vi "MeasureSignals.vi"(6 "Path":path, 8 "error in (no error)":errorcluster caption="Error in", 11 "DevicesAndSignals":T1) -> (0 "error out":errorcluster caption="Error out", 3 "DevicesAndSignals":T1)   [LabVIEW 2016]
doc: "Use this VI to interactively choose signals you want to measure and visualize or save.\n\nDevicesAndSignals: Cluster consisting of an array of devices and an array of all signals you want to measure\nPath: Complete path and name of the file to save measurement values in."
uses:
  <vilib>/Utility/error.llb/DialogType.ctl
panel:
  in  "cmdSaveOnOff":bool
  out "lbDataFile":string
  in  "cmdExit":bool
  in  "Signals":i32(listbox)
  out "Signalverlaufsdiagramm":waveform(dbl)[](graph)
  in  "cmdStop":bool
  in  "cmdStart":bool
  # "Save measurement data"
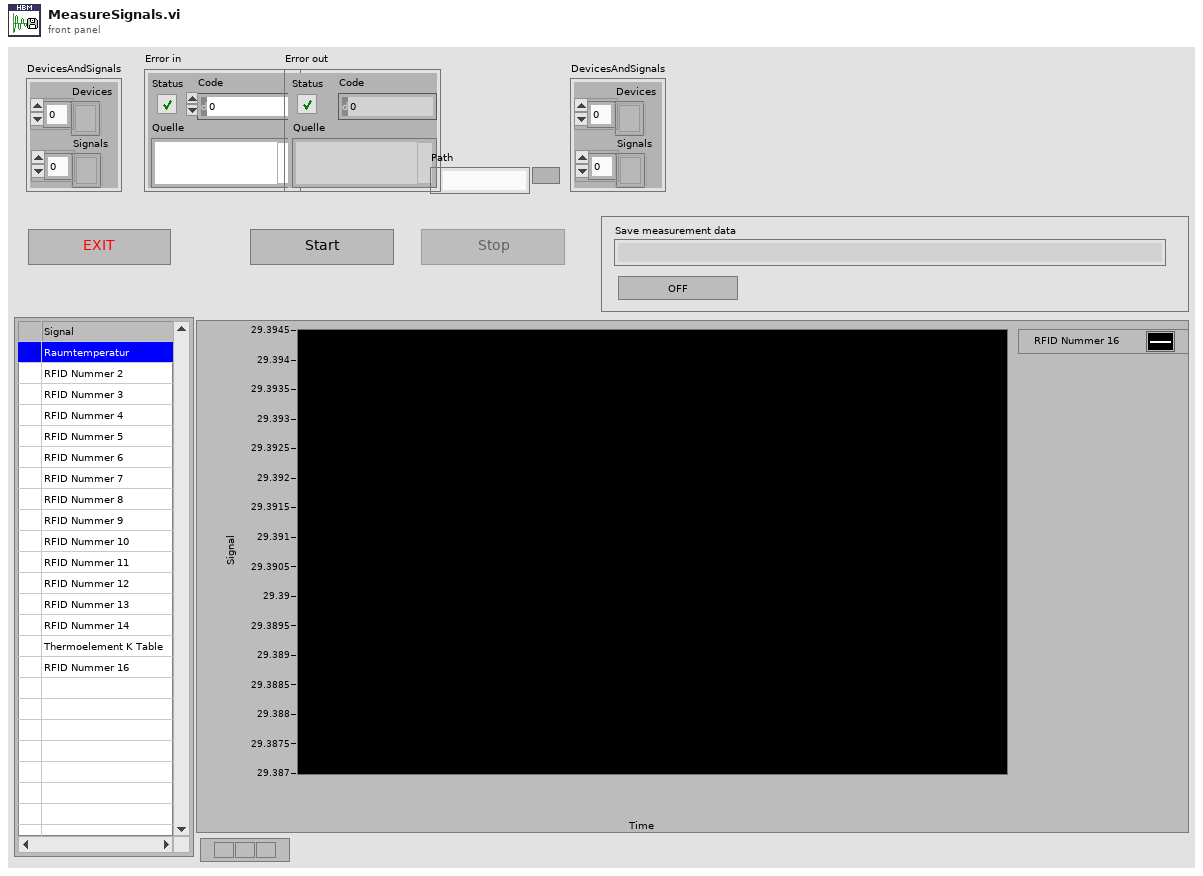
[diagram p1: front panel]
types:
  T1 = cluster{"Devices":refnum<k24>[], "Signals":refnum<k24>[]}
  T2 = enum16{"open", "open or create", "create or replace", "create", "open (read-only)"}
  T3 = cluster{"MeasData":waveform(dbl)[], "State":enum16{"Data", "Exit"}}
  T4 = enum16{"Initialize", "Exit", "DAQ_Start", "DAQ_Stop"}
  T5 = enum16{"Idle", "DAQ_Initialize", "DAQ_Start", "DAQ_Read", "DAQ_Stop", "Exit"}
  T6 = typedef "DialogType.ctl" = u16
  T7 = enum8{"Enabled", "Disabled", "Disabled and Grayed Out"}
  T8 = typedef "LVPoint32TypeDef.ctl" = cluster{"Horizontal":i32, "Vertical":i32}
  T9 = typedef "LVRowAndColumnTypeDef.ctl" = cluster{"Row":i32, "Column":i32}
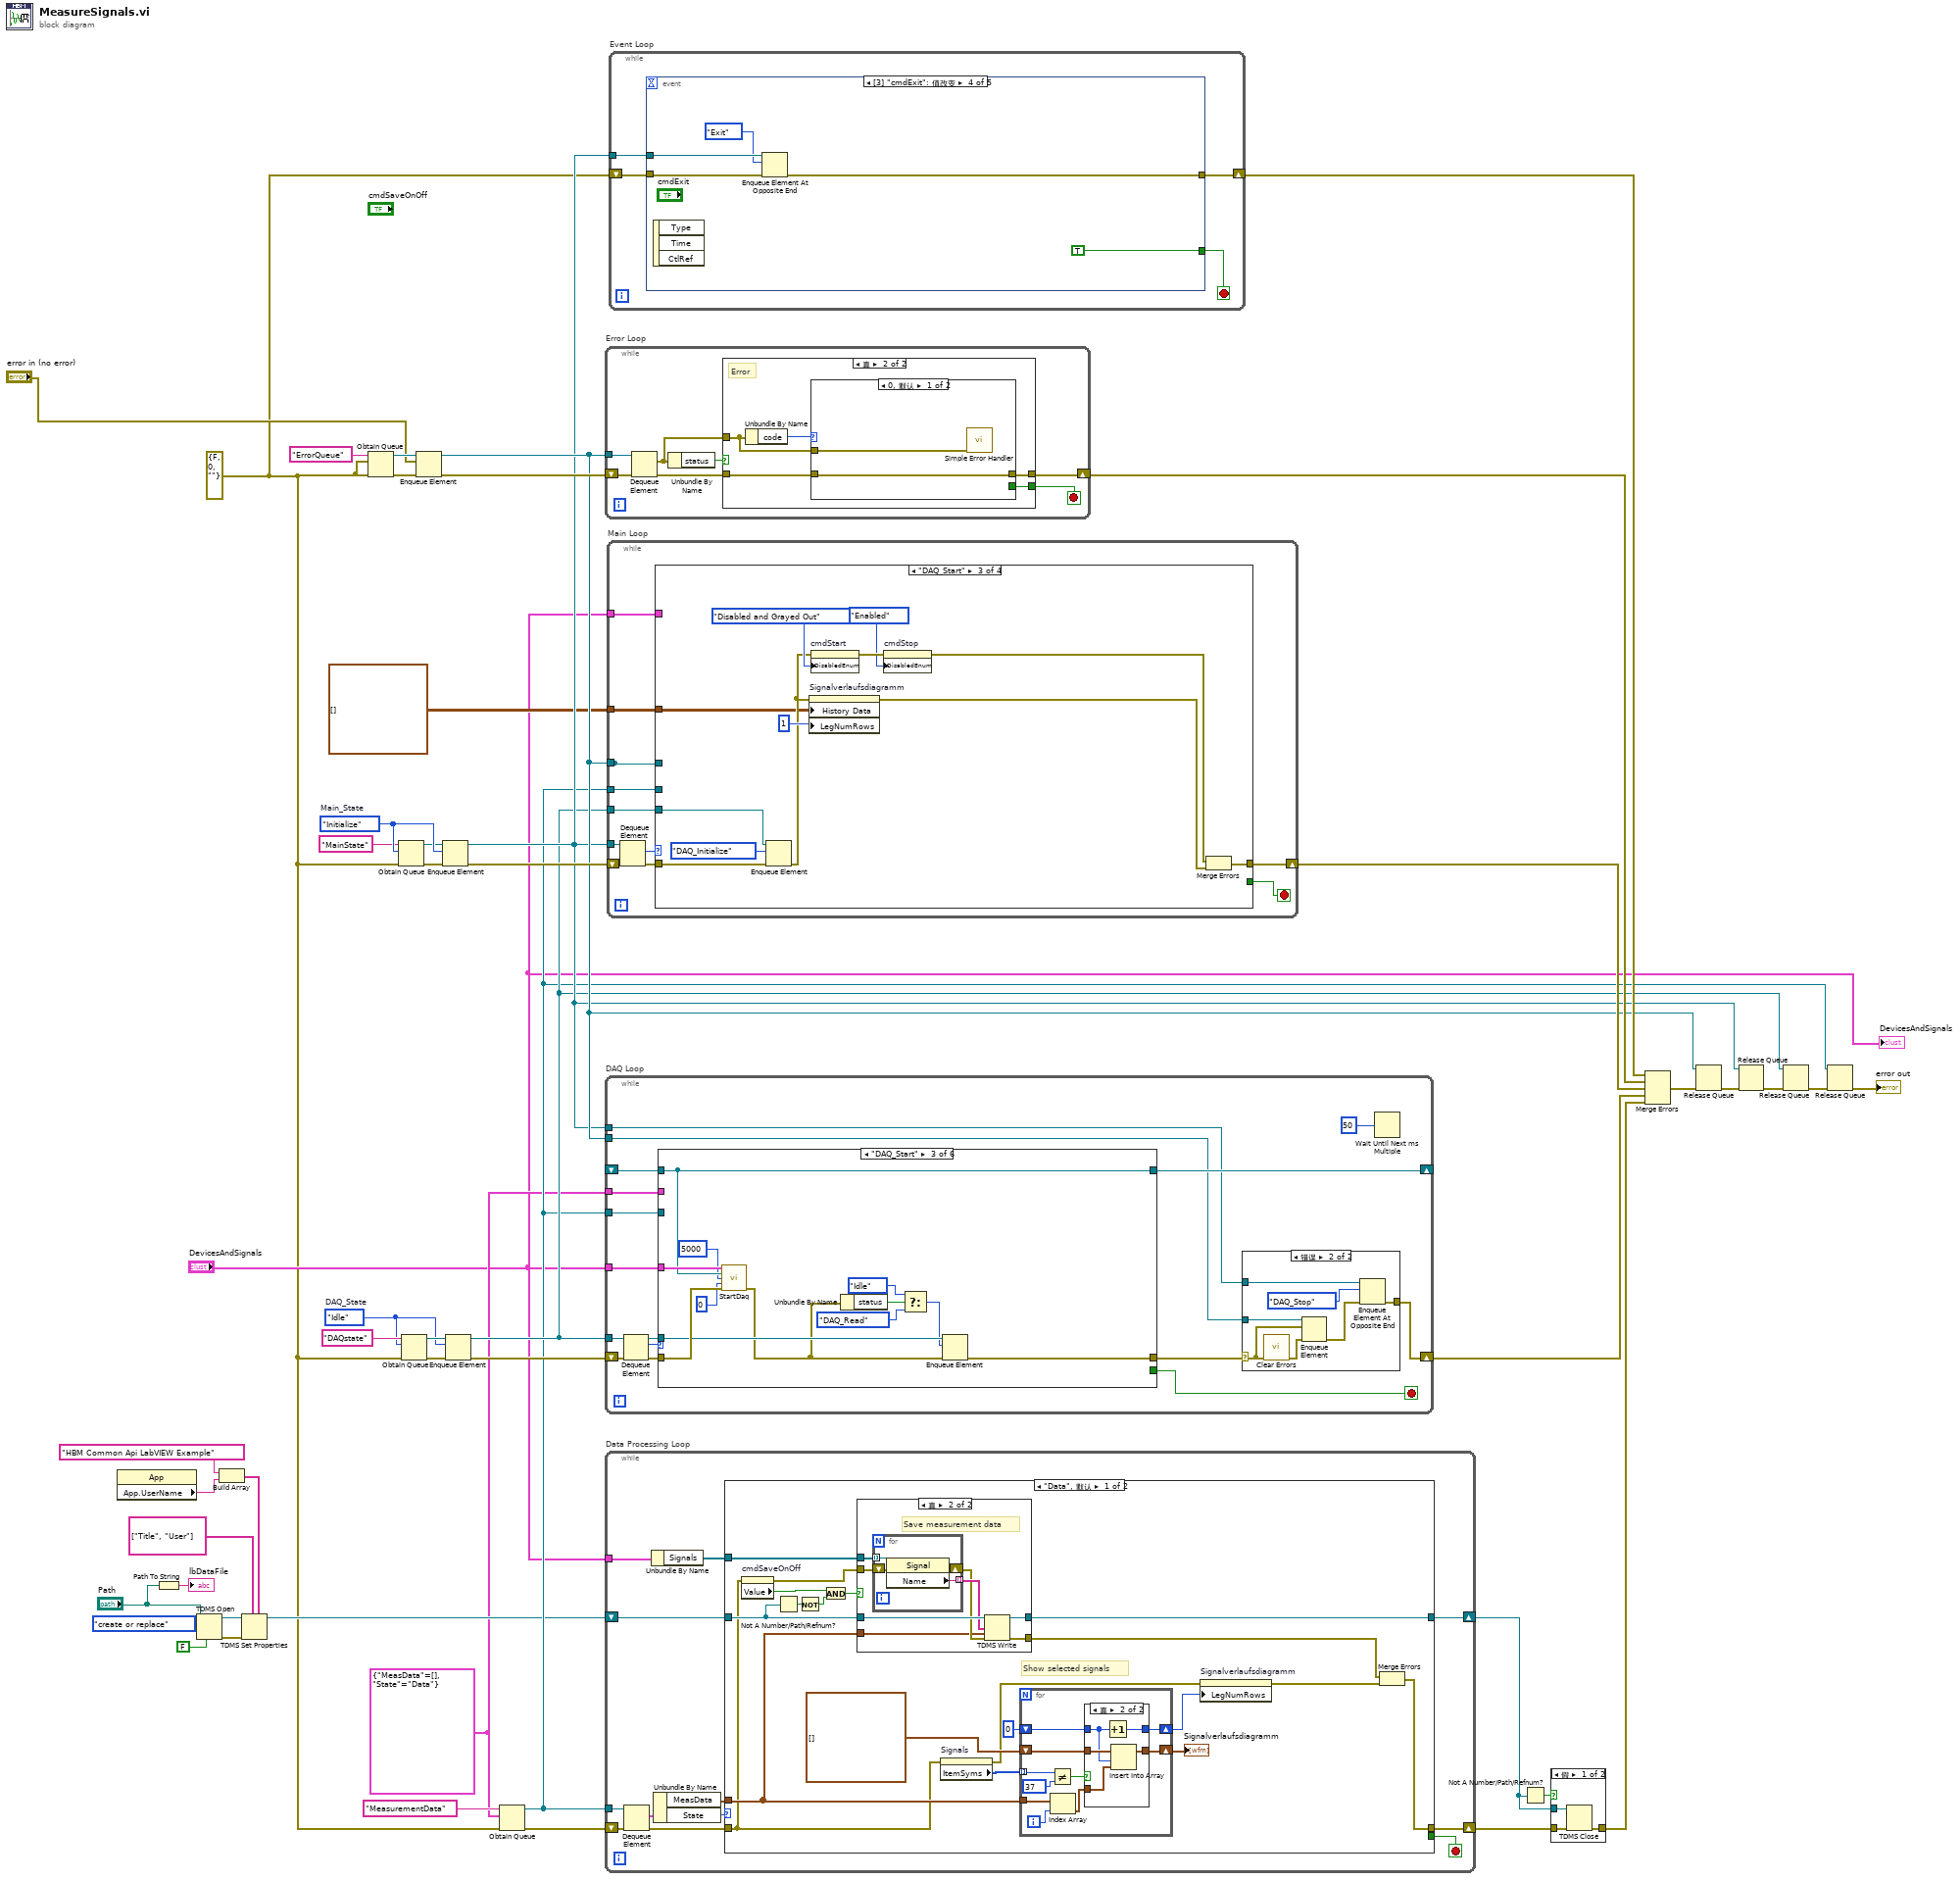
[diagram p0: block diagram]
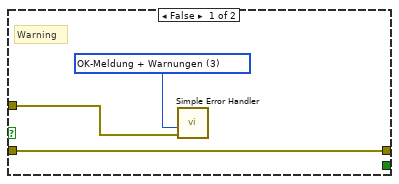
[diagram p3: hidden frame]
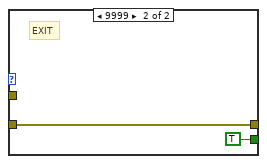
[diagram p4: hidden frame]
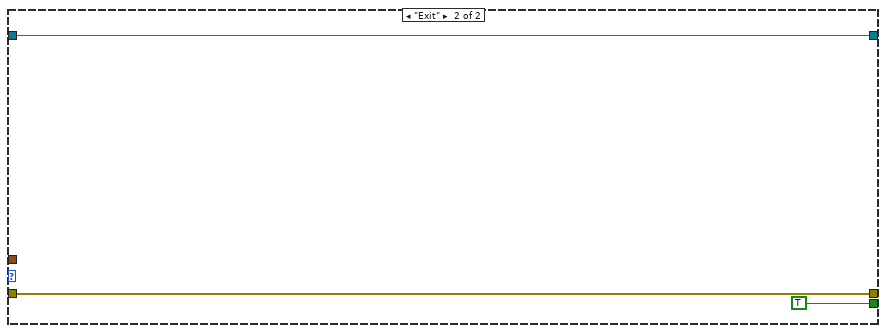
[diagram p7: hidden frame]
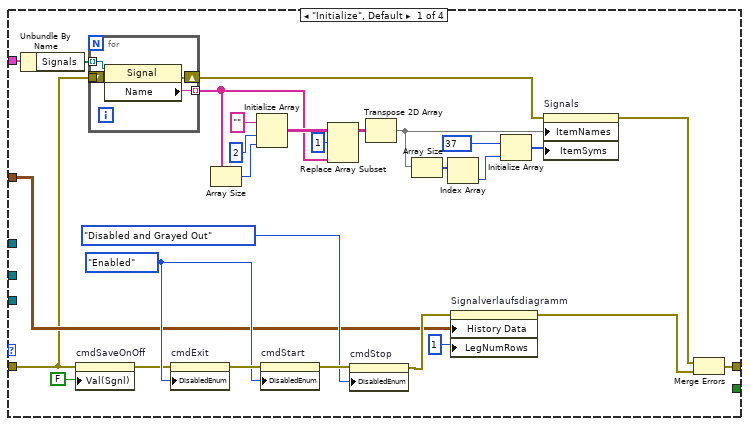
[diagram p8: hidden frame]
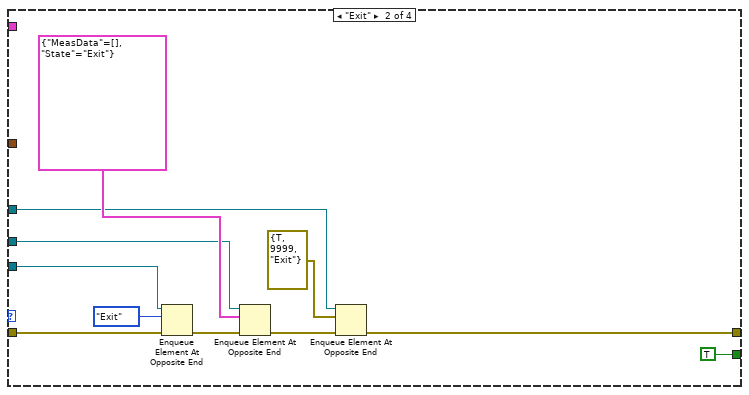
[diagram p9: hidden frame]
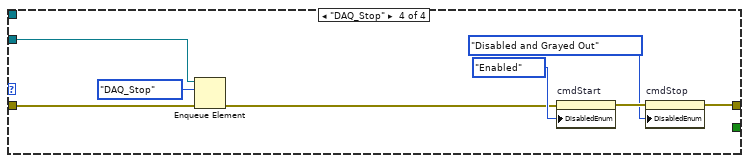
[diagram p10: hidden frame]
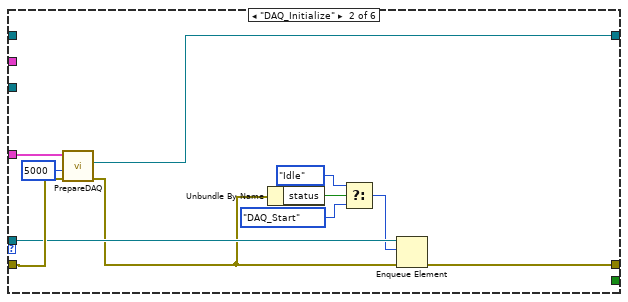
[diagram p13: hidden frame]
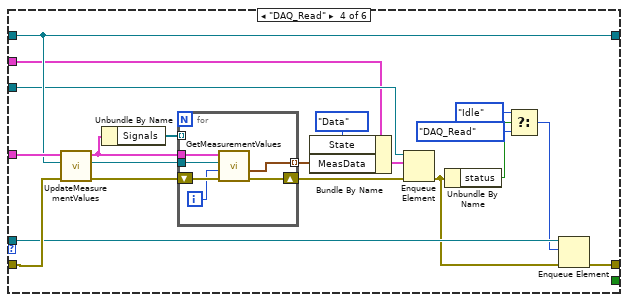
[diagram p14: hidden frame]
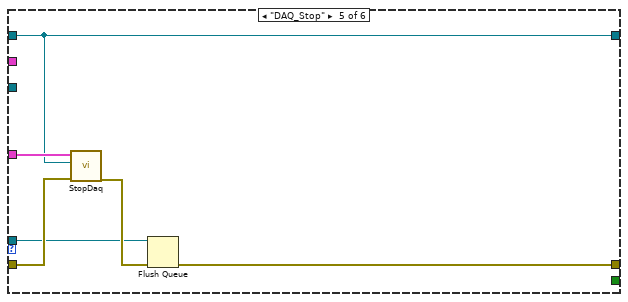
[diagram p15: hidden frame]
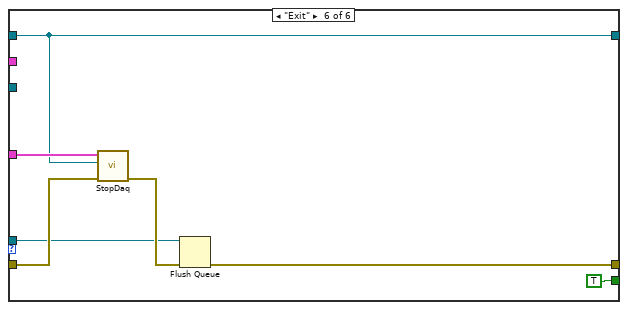
[diagram p16: hidden frame]
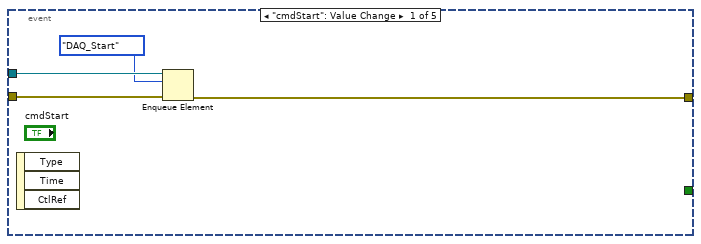
[diagram p17: hidden frame]
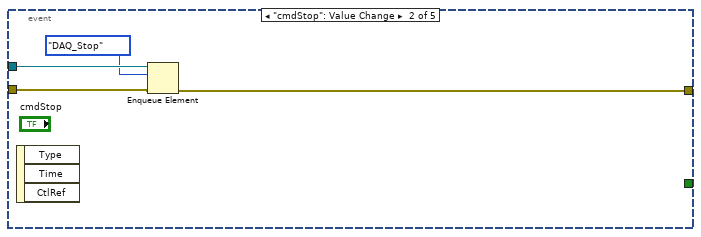
[diagram p18: hidden frame]
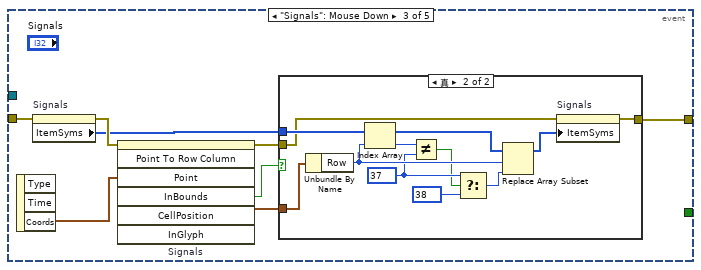
[diagram p19: hidden frame]
diagram:
  w1 = errorcluster {"status"=FALSE, "code"=0, "source"=""} ("Fehler (Eingang, kein Fehler)")
  w11 = T3 {"MeasData"=[], "State"=enum."Data"} ("Element")
  w45 = T4."Initialize"  # Main_State
  w46 = T5."Idle"  # DAQ_State
  n1 = property class="App"() -> ("App.UserName"=w17:string)  [unwired: 2 in, 2 out]
  n2 = Path To String(path="Path") -> (string=→"lbDataFile":string)
  n3 = TDMS Open(6:FALSE ("Pufferung deaktivieren? (T)"), 10:T2."create or replace" ("Operation (0:Öffnen)"), 11:"Path") -> (0:w19:errorcluster, 3:w13:refnum<k34>)  [unwired: 4 in]
  n4 = Build Array("HBM Common Api LabVIEW Example", w17) -> (w16:string[])
  n5 = TDMS Set Properties(5:w16, 7:string[] ["Title", "User"] ("property names"), 8:w19, 11:w13) -> (3:w12:refnum<k34>)  [unwired: 2 in, 3 out]
  n6 = Obtain Queue(name (unnamed)="ErrorQueue" ("Name (unbenannt)"), element data type=w1, error in (no error)=w1) -> (queue out=w37:refnum<queue>, error out=w38:errorcluster)  [unwired: 2 in, 1 out]
  n7 = Obtain Queue(name (unnamed)="MainState" ("Name (unbenannt)"), element data type=w45, error in (no error)=w1) -> (queue out=w44:refnum<queue>, error out=w43:errorcluster)  [unwired: 2 in, 1 out]
  n8 = Obtain Queue(name (unnamed)="DAQstate" ("Name (unbenannt)"), element data type=w46, error in (no error)=w1) -> (queue out=w47:refnum<queue>, error out=w48:errorcluster)  [unwired: 2 in, 1 out]
  n9 = Enqueue Element(queue=w37, element="error in (no error)", error in (no error)=w38) -> (queue out=w24:refnum<queue>, error out=w36:errorcluster)  [unwired: 1 in, 1 out]
  n10 = Enqueue Element(queue=w44, element=w45, error in (no error)=w43) -> (queue out=w23:refnum<queue>, error out=w41:errorcluster)  [unwired: 1 in, 1 out]
  n11 = Enqueue Element(queue=w47, element=w46, error in (no error)=w48) -> (queue out=w22:refnum<queue>, error out=w35:errorcluster)  [unwired: 1 in, 1 out]
  n12 = Obtain Queue(name (unnamed)="MeasurementData" ("Name (unbenannt)"), element data type=w11, error in (no error)=w1) -> (queue out=w21:refnum<queue>, error out=w34:errorcluster)  [unwired: 2 in, 1 out]
  n13 = while "Error Loop" {
    tunnel: w24 -> [w56]
    shift-right: [w50] -> w32
    shift-left: w36 -> [w52]
    stop <- w53 stop-if-true
    n14 = Dequeue Element(queue=w56, error in (no error)=w52) -> (element=w54:errorcluster, error out=w51:errorcluster)  [unwired: 1 in, 2 out]
    n15 = Unbundle By Name(w54) -> ("status"=w55:bool)
    n16 = case "Case-Struktur" shown="真" w55 {
      tunnel: w54 -> [w59 w62]
      tunnel: [_ w63] -> w53
      tunnel: w51 -> [w57 w61]
      tunnel: [w57 w60] -> w50
      frame False {
        w58 = T6 3 items=["Kein Dialog", "OK-Meldung", "Dialog zum Fortsetzen oder Anhalten", "OK-Meldung + Warnungen", "Weiter/Stopp + Warnung"] ("type of dialog (OK msg:1)")
        # "Warning"
        n17 = call <vilib>:"Simple Error Handler.vi"("type of dialog (OK msg:1)"=w58, "error in (no error)"=w59) -> ()  [unwired: 3 in, 5 out]
      }
      frame True {
        # "Error"
        n18 = Unbundle By Name(w62) -> ("code"=w64:i32)
        n19 = case shown="0, 默认" w64 {
          tunnel: [_ TRUE] -> w63
          tunnel: w62 -> [w66 _]
          tunnel: w61 -> [w65 w67]
          tunnel: [w65 w67] -> w60
          frame 0, Default {
            n20 = call <vilib>:"Simple Error Handler.vi"("error in (no error)"=w66) -> ()  [unwired: 4 in, 5 out]
          }
          frame 9999 {
            # "EXIT"
          }
        }
      }
    }
  }
  n21 = while "DAQ Loop" {
    tunnel: w22 -> [w84]
    tunnel: "DevicesAndSignals" -> [w82]
    shift-right: [w81] -> _
    shift-left: _ -> [w78]
    shift-right: [w72] -> w30
    shift-left: w35 -> [w80]
    tunnel: w21 -> [w75]
    tunnel: w11 -> [w74]
    tunnel: w24 -> [w73]
    tunnel: w23 -> [w71]
    stop <- w76 stop-if-true
    n22 = Dequeue Element(queue=w84, error in (no error)=w80) -> (queue out=w77:refnum<queue>, element=w83:T5, error out=w79:errorcluster)  [unwired: 1 in, 1 out]
    n23 = case shown="\"DAQ_Start\"" w83 {
      tunnel: w82 -> [_ w105 w117 w137 w148 w156]
      tunnel: [w94 w103 w116 w131 w144 w150] -> w81
      tunnel: w79 -> [w93 w104 w115 w132 w149 w155]
      tunnel: w78 -> [w94 _ w116 w131 w144 w150]
      tunnel: [w93 w98 w113 w122 w147 w151] -> w69
      tunnel: w77 -> [_ w99 w114 w121 w145 w152]
      tunnel: [_ _ _ _ _ TRUE] -> w76
      tunnel: w75 -> [_ _ _ w129 _ _]
      tunnel: w74 -> [_ _ _ w128 _ _]
      frame "Idle", Default {
      }
      frame "DAQ_Initialize" {
        n24 = call "PrepareDAQ.vi"("Error in"=w104, "BufferTimeout"=5000, "DevicesAndSignals"=w105) -> ("Error out"=w97:errorcluster, "DaqMeasurement"=w103:refnum<k24>)  [unwired: 6 in, 1 out]
        n25 = Unbundle By Name(w97) -> ("status"=w100:bool)
        n26 = Select(t=T5."Idle" ("Element"), s=w100, f=T5."DAQ_Start" ("Element")) -> (s? t:f=w96:T5)
        n27 = Enqueue Element(queue=w99, element=w96, error in (no error)=w97) -> (error out=w98:errorcluster)  [unwired: 1 in, 2 out]
      }
      frame "DAQ_Start" {
        n28 = call "StartDaq.vi"("DevicesAndSignals"=w117, "DaqMeasurement"=w116, "SyncTimeout"=5000, "AcquisitionMode"=0, "Error in"=w115) -> ("Error out"=w108:errorcluster)  [unwired: 7 in, 3 out]
        n29 = Unbundle By Name(w108) -> ("status"=w110:bool)
        n30 = Select(t=T5."Idle" ("Element"), s=w110, f=T5."DAQ_Read" ("Element")) -> (s? t:f=w109:T5)
        n31 = Enqueue Element(queue=w114, element=w109, error in (no error)=w108) -> (error out=w113:errorcluster)  [unwired: 1 in, 2 out]
      }
      frame "DAQ_Read" {
        n32 = call "UpdateMeasurementValues.vi"("Error in"=w132, "DaqMeasurement"=w131, "DevicesAndSignals"=w137) -> ("Error out"=w135:errorcluster, "DaqMeasurement"=w136:refnum<k24>, "DevicesAndSignals"=w134:T1)  [unwired: 6 in]
        n33 = Unbundle By Name(w134) -> ("Signals"=w133:refnum<k24>[])
        n34 = for {
          tunnel: w134 -> [w143]
          tunnel: w136 -> [w142]
          shift-right: [w141] -> w130
          shift-left: w135 -> [w140]
          tunnel: w133 -> [_] mode=indexing
          tunnel: [w138] -> w126 mode=indexing
          i -> [w139]
          n35 = call "GetMeasurementValues.vi"("Error in"=w140, "Index"=w139, "DaqMeasurement"=w142, "DevicesAndSignals"=w143) -> ("Error out"=w141:errorcluster, "Waveform"=w138:waveform(dbl))  [unwired: 4 in, 2 out]
        }
        n36 = Bundle By Name(cluster=w128, "State"=enum16{"Data", "Exit"}."Data", "MeasData"=w126) -> (w127:T3)
        n37 = Enqueue Element(queue=w129, element=w127, error in (no error)=w130) -> (error out=w118:errorcluster)  [unwired: 1 in, 2 out]
        n38 = Unbundle By Name(w118) -> ("status"=w119:bool)
        n39 = Select(t=T5."Idle" ("Element"), s=w119, f=T5."DAQ_Read" ("Element")) -> (s? t:f=w120:T5)
        n40 = Enqueue Element(queue=w121, element=w120, error in (no error)=w118) -> (error out=w122:errorcluster)  [unwired: 1 in, 2 out]
      }
      frame "DAQ_Stop" {
        n41 = call "StopDaq.vi"("Error in"=w149, "DaqMeasurement"=w144, "DevicesAndSignals"=w148) -> ("Error out"=w146:errorcluster)  [unwired: 7 in, 1 out]
        n42 = Flush Queue(queue=w145, error in (no error)=w146) -> (error out=w147:errorcluster)  [unwired: 2 out]
      }
      frame "Exit" {
        n43 = call "StopDaq.vi"("Error in"=w155, "DaqMeasurement"=w150, "DevicesAndSignals"=w156) -> ("Error out"=w153:errorcluster)  [unwired: 7 in, 1 out]
        n44 = Flush Queue(queue=w152, error in (no error)=w153) -> (error out=w151:errorcluster)  [unwired: 2 out]
      }
    }
    n45 = case shown="错误" w69 {
      selector: w69 -> [w85 w86]
      tunnel: w73 -> [_ w92]
      tunnel: [w85 w88] -> w72
      tunnel: w71 -> [_ w90]
      frame No Error {
      }
      frame Error {
        n46 = call <vilib>:"Clear Errors.vi"("error in (no error)"=w86) -> ("error out"=w91:errorcluster)  [unwired: 5 in, 1 out]
        n47 = Enqueue Element(queue=w92, element=w86, error in (no error)=w91) -> (error out=w89:errorcluster)  [unwired: 1 in, 2 out]
        n48 = Enqueue Element At Opposite End(queue=w90, element=T4."DAQ_Stop" ("Element"), error in (no error)=w89) -> (error out=w88:errorcluster)  [unwired: 1 in, 2 out]
      }
    }
    n49 = Wait Until Next ms Multiple(millisecond multiple=u32 50 ("Vielfache von ms")) -> ()  [unwired: 1 out]
  }
  n50 = while "Data Processing Loop" {
    tunnel: "DevicesAndSignals" -> [w160]
    tunnel: w21 -> [w168]
    shift-right: [w163] -> w5
    shift-left: w34 -> [w165]
    shift-right: [w161] -> w7
    shift-left: w12 -> [w162]
    stop <- w166 stop-if-true
    n51 = Dequeue Element(queue=w168, error in (no error)=w165) -> (element=w158:T3, error out=w164:errorcluster)  [unwired: 1 in, 2 out]
    n52 = Unbundle By Name(w160) -> ("Signals"=w159:refnum<k24>[])
    n53 = Unbundle By Name(w158) -> ("MeasData"=w157:waveform(dbl)[], "State"=w167:enum16{"Data", "Exit"})
    n54 = case shown="\"Data\", 默认" w167 {
      tunnel: [_ TRUE] -> w166
      tunnel: w164 -> [w171 w220]
      tunnel: [w173 w220] -> w163
      tunnel: w162 -> [w178 w219]
      tunnel: [w187 w219] -> w161
      tunnel: w159 -> [w181 _]
      tunnel: w157 -> [w180 _]
      frame "Data", Default {
        # "Show selected signals"
        n55 = property on="cmdSaveOnOff" class="Bool (严格)"(error in=w171) -> (error out=w170:errorcluster, "Value"=w169:bool)  [unwired: 1 in, 1 out]
        n56 = Not A Number/Path/Refnum?(number/path/refnum=w178) -> (NaN/Path/Refnum?=w177:bool)
        n57 = Not(x=w177) -> (.not. x?=w176:bool)
        n58 = And(x=w169, y=w176) -> (x .and. y?=w175:bool)
        n59 = case "Case-Struktur" shown="真" w175 {
          tunnel: w178 -> [w189 w197]
          tunnel: [w189 w196] -> w187
          tunnel: w181 -> [_ w193]
          tunnel: w180 -> [_ w192]
          tunnel: w170 -> [w188 w191]
          tunnel: [w188 w190] -> w174
          frame False {
          }
          frame True {
            # "Save measurement data"
            n60 = for {
              tunnel: w193 -> [w201] mode=indexing
              tunnel: [w200] -> w195 mode=indexing
              shift-right: [w198] -> w194
              shift-left: w191 -> [w199]
              n61 = property on="Eigenschaftsknoten" class="Signal"(reference=w201, error in=w199) -> (error out=w198:errorcluster, "Name"=w200:string)  [unwired: 1 out]
            }
            n62 = TDMS Write(0:w197, 7:w195, 9:w192, 11:w194) -> (4:w196:refnum<k34>, 15:w190:errorcluster)  [unwired: 2 in, 2 out]
          }
        }
        n63 = property on="Signals" class="MCListbox (严格)"(error in=w171) -> (error out=w179:errorcluster, "ItemSyms"=w186:i32[])  [unwired: 1 in, 1 out]
        n64 = for {
          tunnel: w180 -> [w211]
          tunnel: w186 -> [w209] mode=indexing
          shift-right: [w205] -> w183
          shift-left: waveform(dbl)[] [] -> [w204]
          shift-right: [w202] -> w182
          shift-left: u32 0 -> [w203]
          i -> [w208]
          n65 = Not Equal?(x=w209, y=37) -> (x != y?=w206:bool)
          n66 = Index Array(array=w211, index=w208) -> (element=w207:waveform(dbl))
          n67 = case shown="真" w206 {
            tunnel: [w213 w218] -> w205
            tunnel: w204 -> [w213 w217]
            tunnel: [w212 w215] -> w202
            tunnel: w207 -> [_ w216]
            tunnel: w203 -> [w212 w214]
            frame False {
            }
            frame True {
              n68 = Increment(x=w214) -> (x+1=w215:u32)
              n69 = Insert Into Array(array=w217, index=w214, new element=w216) -> (w218:waveform(dbl)[])
            }
          }
        }
        "Signalverlaufsdiagramm" <- w183
        n70 = property on="Signalverlaufsdiagramm" class="WFChart (严格)"(error in=w179, "LegNumRows"=w182) -> (error out=w172:errorcluster)  [unwired: 1 in, 1 out]
        n71 = Merge Errors(w174, w172) -> (w173:errorcluster)
      }
      frame "Exit" {
      }
    }
  }
  n72 = while "Main Loop" {
    shift-right: [w226] -> w33
    shift-left: w41 -> [w232]
    tunnel: w23 -> [w231]
    tunnel: w22 -> [w228]
    tunnel: w21 -> [w225]
    tunnel: [w224] -> _
    tunnel: w24 -> [w224]
    tunnel: "DevicesAndSignals" -> [w223]
    tunnel: waveform(dbl)[][] [] ("Historiendaten") -> [w222]
    stop <- w227 stop-if-true
    n73 = Dequeue Element(queue=w231, error in (no error)=w232) -> (element=w230:T4, error out=w229:errorcluster)  [unwired: 1 in, 2 out]
    n74 = case shown="\"DAQ_Start\"" w230 {
      tunnel: w229 -> [w235 w273 w286 w294]
      tunnel: w228 -> [_ w274 w285 w293]
      tunnel: [_ TRUE _ _] -> w227
      tunnel: [w241 w266 w279 w289] -> w226
      tunnel: w225 -> [_ w270 _ _]
      tunnel: w224 -> [_ w268 _ _]
      tunnel: w223 -> [w256 _ _ _]
      tunnel: w222 -> [w237 _ w276 _]
      frame "Initialize", Default {
        w258 = T7."Enabled" ("Deaktiviert")
        n75 = Unbundle By Name(w256) -> ("Signals"=w255:refnum<k24>[])
        n76 = property on="cmdSaveOnOff" class="Bool (严格)"(error in=w235, "Val(Sgnl)"=FALSE ("Wert (signalisierend)")) -> (error out=w234:errorcluster)  [unwired: 1 in, 1 out]
        n77 = for {
          tunnel: [w264] -> w245 mode=indexing
          tunnel: w235 -> [w263]
          tunnel: w255 -> [w262] mode=indexing
          shift-right: [w261] -> w242
          shift-left: _ -> [_]
          n78 = property on="Eigenschaftsknoten" class="Signal"(reference=w262, error in=w263) -> (error out=w261:errorcluster, "Name"=w264:string)  [unwired: 1 out]
        }
        n79 = property on="cmdExit" class="Bool"(error in=w234, "DisabledEnum"=w258) -> (error out=w260:errorcluster)  [unwired: 1 in, 1 out]
        n80 = Array Size(array=w245) -> (size(s)=w249:i32)
        n81 = Initialize Array("" ("Element"), 2 ("Dimension"), w249) -> (w253:string[][])
        n82 = property on="cmdStart" class="Bool"(error in=w260, "DisabledEnum"=w258) -> (error out=w259:errorcluster)  [unwired: 1 in, 1 out]
        n83 = Replace Array Subset(array=w253, new element=w245, index (row)=1 ("Index (Zeile)")) -> (w251:string[][])  [unwired: 1 in]
        n84 = property on="cmdStop" class="Bool"(error in=w259, "DisabledEnum"=T7."Disabled and Grayed Out" ("Deaktiviert")) -> (error out=w239:errorcluster)  [unwired: 1 in, 1 out]
        n85 = Transpose 2D Array(2D array=w251) -> (transposed array=w244:string[][])
        n86 = Array Size(array=w244) -> (size(s)=w248:i32[])
        n87 = Index Array(array=w248) -> (element=w247:i32)  [unwired: 1 in]
        n88 = property on="Signalverlaufsdiagramm" class="WFChart (严格)"(error in=w239, "History Data"=w237, "LegNumRows"=u32 1 ("Legende:Zeilenanzahl")) -> (error out=w238:errorcluster)  [unwired: 1 in, 1 out]
        n89 = Initialize Array(37, w247) -> (w243:i32[])
        n90 = property on="Signals" class="MCListbox (严格)"(error in=w242, "ItemNames"=w244, "ItemSyms"=w243) -> (error out=w240:errorcluster)  [unwired: 1 in, 1 out]
        n91 = Merge Errors(w240, w238) -> (w241:errorcluster)
      }
      frame "Exit" {
        n92 = Enqueue Element At Opposite End(queue=w274, element=T5."Exit" ("Element"), error in (no error)=w273) -> (error out=w269:errorcluster)  [unwired: 1 in, 2 out]
        n93 = Enqueue Element At Opposite End(queue=w270, element=T3 {"MeasData"=[], "State"=enum."Exit"} ("Element"), error in (no error)=w269) -> (error out=w267:errorcluster)  [unwired: 1 in, 2 out]
        n94 = Enqueue Element At Opposite End(queue=w268, element=errorcluster {"status"=TRUE, "code"=9999, "source"="Exit"} ("Element"), error in (no error)=w267) -> (error out=w266:errorcluster)  [unwired: 1 in, 2 out]
      }
      frame "DAQ_Start" {
        n95 = Enqueue Element(queue=w285, element=T5."DAQ_Initialize" ("Element"), error in (no error)=w286) -> (error out=w280:errorcluster)  [unwired: 1 in, 2 out]
        n96 = property on="Signalverlaufsdiagramm" class="WFChart (严格)"(error in=w280, "History Data"=w276, "LegNumRows"=u32 1 ("Legende:Zeilenanzahl")) -> (error out=w277:errorcluster)  [unwired: 1 in, 1 out]
        n97 = property on="cmdStart" class="Bool"(error in=w280, "DisabledEnum"=T7."Disabled and Grayed Out" ("Deaktiviert")) -> (error out=w284:errorcluster)  [unwired: 1 in, 1 out]
        n98 = property on="cmdStop" class="Bool"(error in=w284, "DisabledEnum"=T7."Enabled" ("Deaktiviert")) -> (error out=w278:errorcluster)  [unwired: 1 in, 1 out]
        n99 = Merge Errors(w278, w277) -> (w279:errorcluster)
      }
      frame "DAQ_Stop" {
        n100 = Enqueue Element(queue=w293, element=T5."DAQ_Stop" ("Element"), error in (no error)=w294) -> (error out=w288:errorcluster)  [unwired: 1 in, 2 out]
        n101 = property on="cmdStart" class="Bool"(error in=w288, "DisabledEnum"=T7."Enabled" ("Deaktiviert")) -> (error out=w292:errorcluster)  [unwired: 1 in, 1 out]
        n102 = property on="cmdStop" class="Bool"(error in=w292, "DisabledEnum"=T7."Disabled and Grayed Out" ("Deaktiviert")) -> (error out=w289:errorcluster)  [unwired: 1 in, 1 out]
      }
    }
  }
  n103 = while "Event Loop" {
    tunnel: w23 -> [w299]
    shift-right: [w296] -> w31
    shift-left: w1 -> [w297]
    stop <- w298 stop-if-true
    n104 = event shown="[3] \"cmdExit\": 值改变" {
      selector: _ -> [_ _ _ _ _]
      dyn-events: _ -> [_ _ _ _ _]
      timeout: _ -> [_ _ _ _ _]
      tunnel: w299 -> [w303 w307 _ w331 w335]
      tunnel: [_ _ _ TRUE TRUE] -> w298
      tunnel: w297 -> [w301 w305 w315 w329 w334]
      tunnel: [w300 w304 w308 w328 _] -> w296
      event "cmdStart": Value Change {
        n105 = event-data() -> ()  [unwired: 1 in, 3 out]
        n106 = Enqueue Element(queue=w303, element=T4."DAQ_Start" ("Element"), error in (no error)=w301) -> (error out=w300:errorcluster)  [unwired: 1 in, 2 out]
      }
      event "cmdStop": Value Change {
        n107 = event-data() -> ()  [unwired: 1 in, 3 out]
        n108 = Enqueue Element(queue=w307, element=T4."DAQ_Stop" ("Element"), error in (no error)=w305) -> (error out=w304:errorcluster)  [unwired: 1 in, 2 out]
      }
      event "Signals": Mouse Down {
        n109 = event-data() -> ("Coords"=w313:T8)  [unwired: 1 in, 2 out]
        n110 = property on="Signals" class="MCListbox (严格)"(error in=w315) -> (error out=w314:errorcluster, "ItemSyms"=w311:i32[])  [unwired: 1 in, 1 out]
        n111 = invoke on="Signals" class="MehrSpaltFeld (strikt)" method="Point To Row Column"(error in=w314, "Point"=w313) -> (error out=w310:errorcluster, "InBounds"=w309:bool, "CellPosition"=w312:T9)  [unwired: 5 in, 4 out]
        n112 = case shown="真" w309 {
          tunnel: w312 -> [_ w321]
          tunnel: w311 -> [_ w320]
          tunnel: w310 -> [w316 w318]
          tunnel: [w316 w317] -> w308
          frame False {
          }
          frame True {
            w323 = 37
            n113 = Unbundle By Name(w321) -> ("Row"=w327:i32)
            n114 = Index Array(array=w320, index=w327) -> (element=w324:i32)
            n115 = Not Equal?(x=w324, y=w323) -> (x != y?=w322:bool)
            n116 = Select(t=w323, s=w322, f=38) -> (s? t:f=w325:i32)
            n117 = Replace Array Subset(array=w320, new element=w325, index=w327) -> (w319:i32[])
            n118 = property on="Signals" class="MCListbox (严格)"(error in=w318, "ItemSyms"=w319) -> (error out=w317:errorcluster)  [unwired: 1 in, 1 out]
          }
        }
      }
      event "cmdExit": Value Change {
        n119 = event-data() -> ()  [unwired: 1 in, 3 out]
        n120 = Enqueue Element At Opposite End(queue=w331, element=T4."Exit" ("Element"), error in (no error)=w329) -> (error out=w328:errorcluster)  [unwired: 1 in, 2 out]
      }
      event Application Instance Close {
        n121 = event-data() -> ()  [unwired: 1 in, 3 out]
        n122 = Enqueue Element At Opposite End(queue=w335, element=T4."Exit" ("Element"), error in (no error)=w334) -> ()  [unwired: 1 in, 3 out]
      }
    }
  }
  n123 = Not A Number/Path/Refnum?(number/path/refnum=w7) -> (NaN/Path/Refnum?=w6:bool)
  n124 = case shown="假" w6 {
    tunnel: w7 -> [w339 _]
    tunnel: w5 -> [w338 w340]
    tunnel: [w337 w340] -> w4
    frame False {
      n125 = TDMS Close(8:w338, 11:w339) -> (0:w337:errorcluster)  [unwired: 1 out]
    }
    frame True {
    }
  }
  n126 = Merge Errors(w31, w32, w33, w30, w4) -> (w26:errorcluster)
  n127 = Release Queue(queue=w24, error in (no error)=w26) -> (error out=w29:errorcluster)  [unwired: 1 in, 2 out]
  n128 = Release Queue(queue=w23, error in (no error)=w29) -> (error out=w28:errorcluster)  [unwired: 1 in, 2 out]
  n129 = Release Queue(queue=w22, error in (no error)=w28) -> (error out=w27:errorcluster)  [unwired: 1 in, 2 out]
  n130 = Release Queue(queue=w21, error in (no error)=w27) -> (error out=→"error out":errorcluster)  [unwired: 1 in, 2 out]
  "DevicesAndSignals" <- "DevicesAndSignals"
